vi "BLE_Module_EOL.vi"(8 "Error In":errorcluster, 9 "DUTBLEMACAddress":string="d8:3b:da:49:e3:cd", 10 "DUTBLEName":string="MyESP32", 11 "VISA resource name":refnum<visa-resource-name>) -> (0 "Error Out":errorcluster, 2 "FAIL":bool, 3 "PASS":bool, 5 "Read Status":string)   [LabVIEW 2025]
doc: "Simple string based state machine with internal error handling.\n\n--------------------\n<Author>\n<Company>"
uses:
  controls/TypeDefReadBuffer.ctl
  controls/BLE_States.ctl
  <vilib>/Utility/error.llb/Trim Whitespace One-Sided.vi
  <vilib>/Instr/_visa.llb/VISA Configure Serial Port (Instr).vi
panel:
  out "read_buffer":T1
  in  "Stop":bool
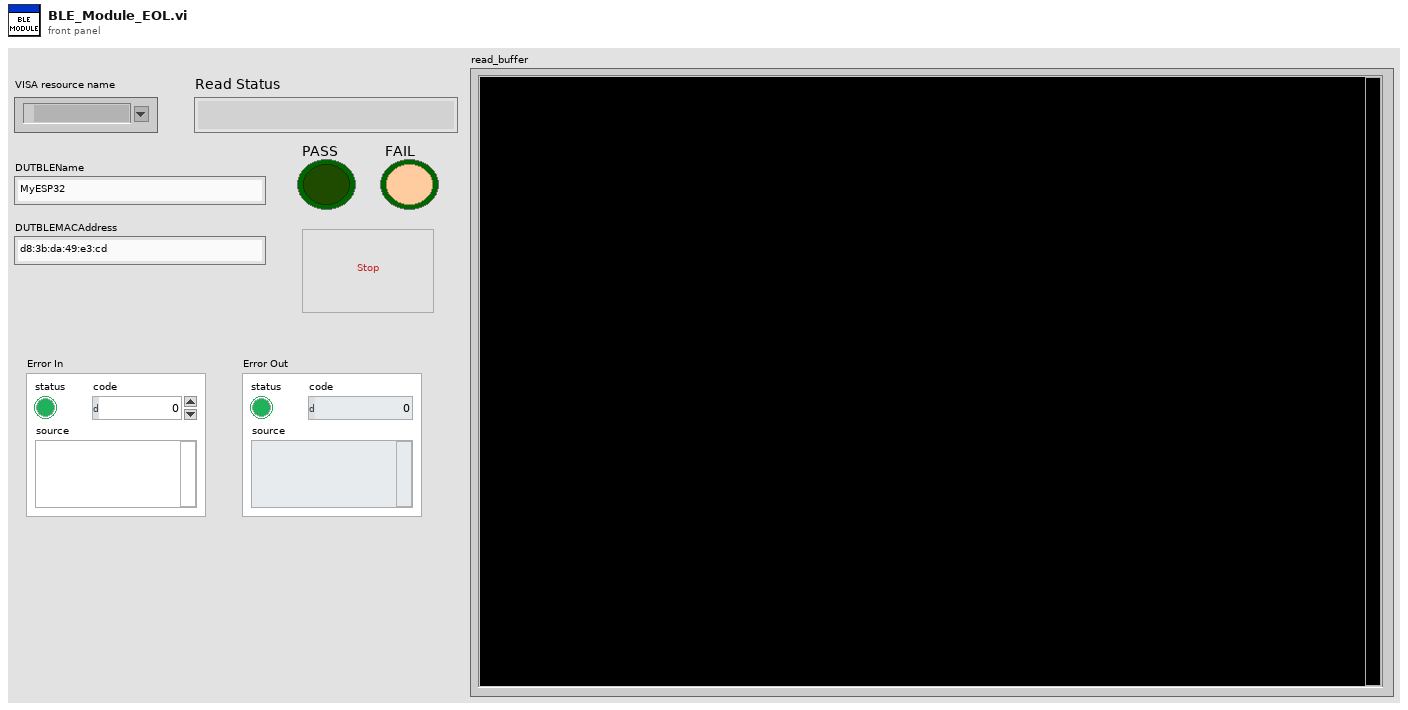
[diagram p1: front panel]
types:
  T1 = typedef "TypeDefReadBuffer.ctl" = string
  T2 = typedef "BLE_States.ctl" = enum16{"Init", "Init_BLE", "DUT_BLE_name", "DUT_BLE_macid", "scan", "ReadSerialContinously", "Disconnect_BLE", "Read_Disconnect_BLE", "Uninit_BLE", "Exit"}
  T3 = cluster{"Message":string, "VISA resource name":refnum<visa-resource-name>}
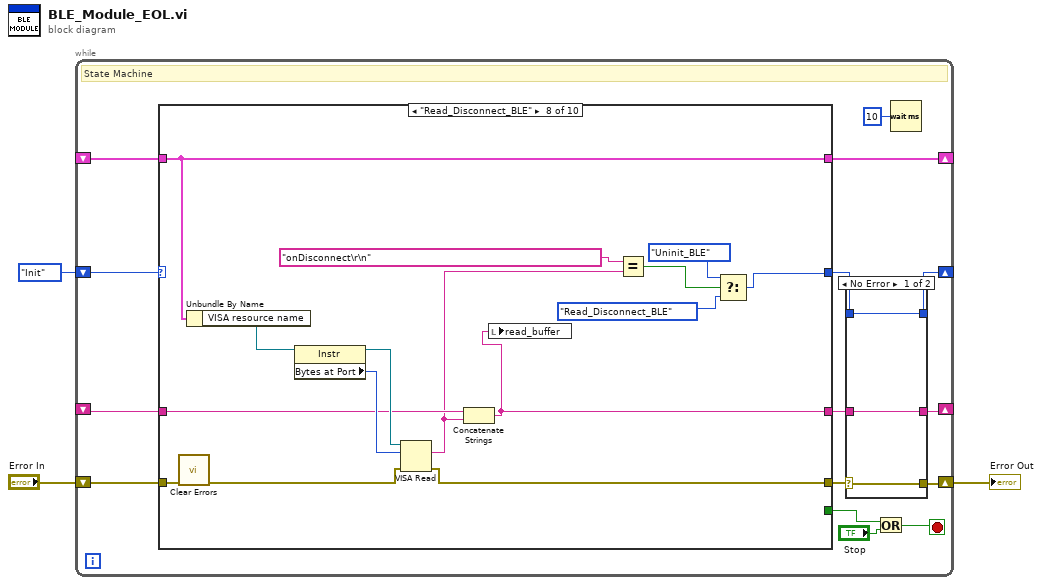
[diagram p0: block diagram]
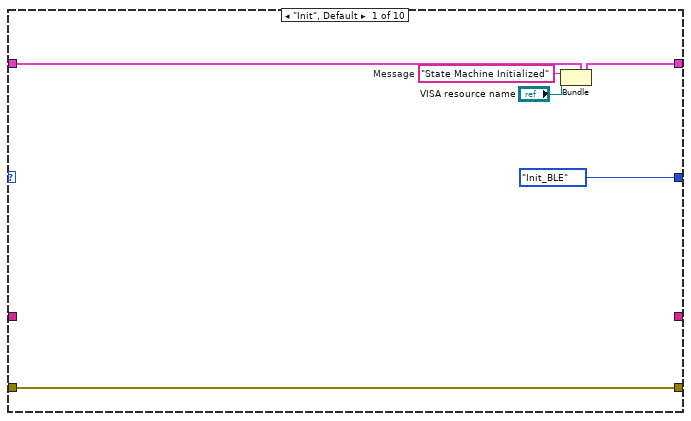
[diagram p2: hidden frame]
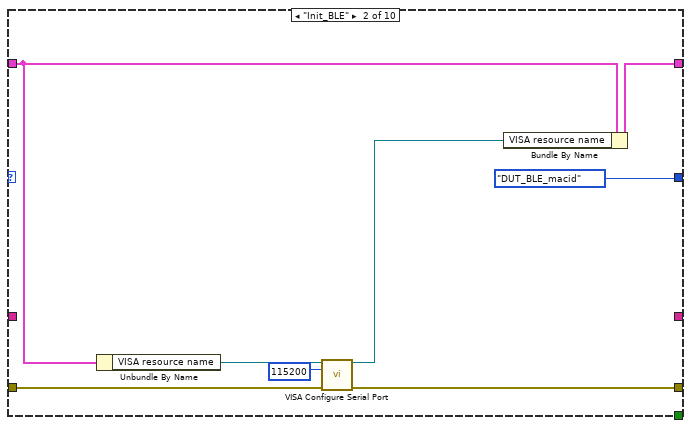
[diagram p3: hidden frame]
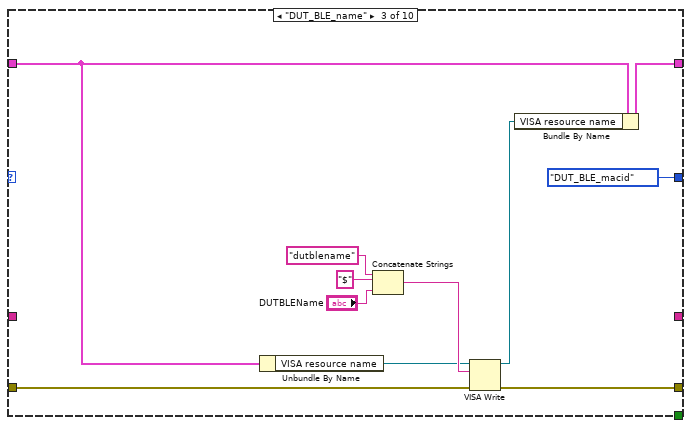
[diagram p4: hidden frame]
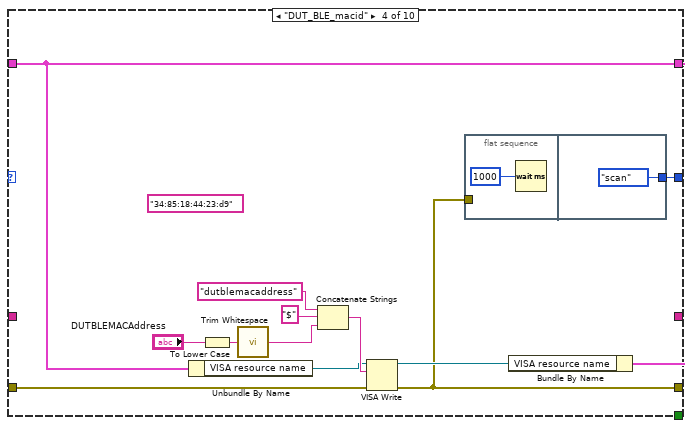
[diagram p5: hidden frame]
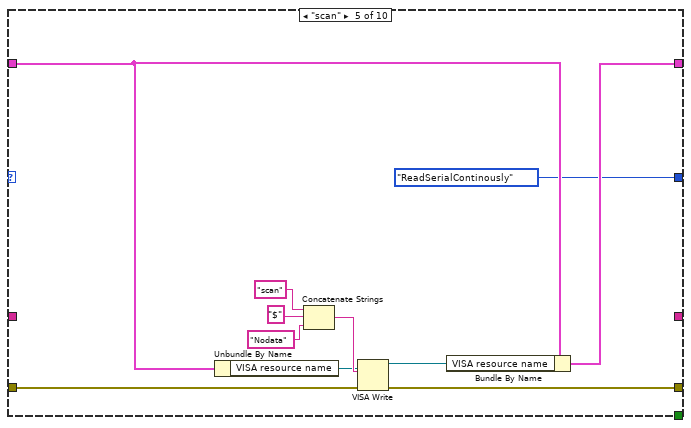
[diagram p6: hidden frame]
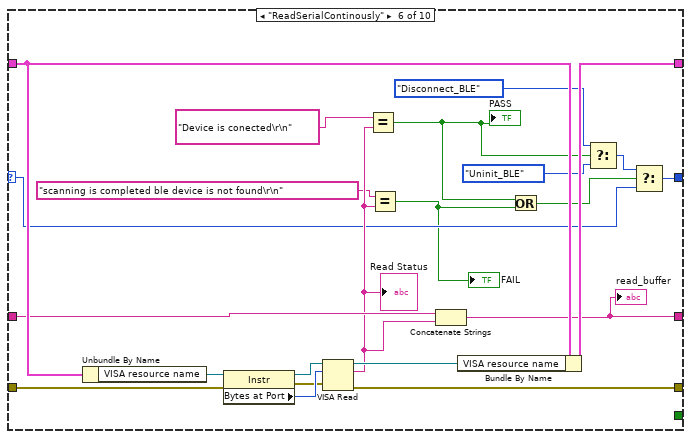
[diagram p7: hidden frame]
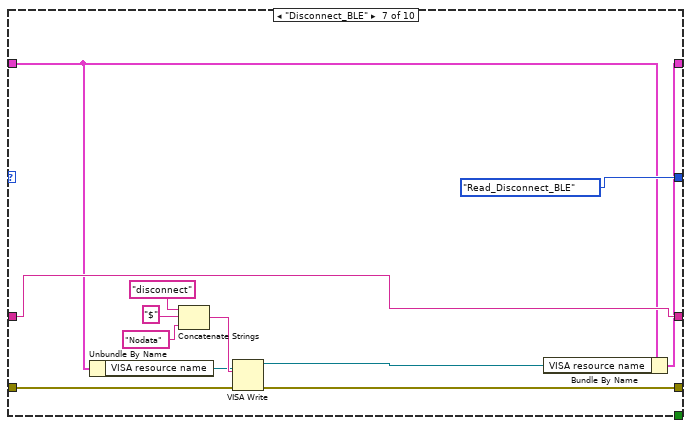
[diagram p8: hidden frame]
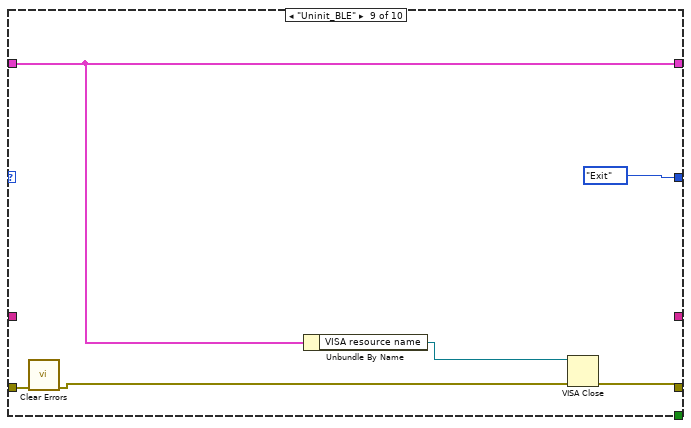
[diagram p9: hidden frame]
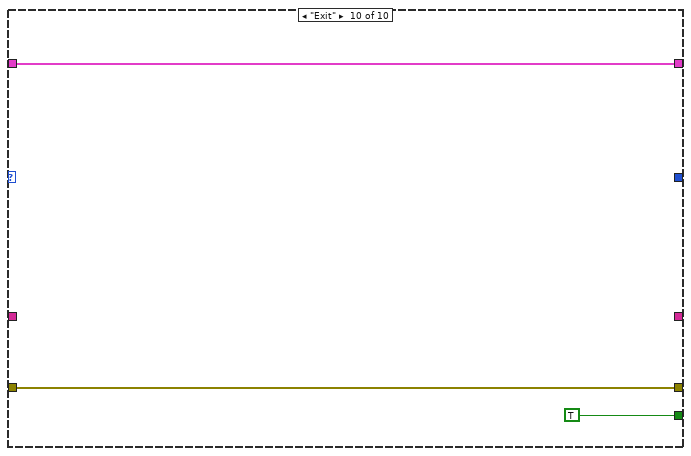
[diagram p10: hidden frame]
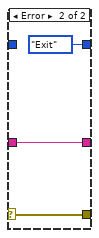
[diagram p11: hidden frame]
diagram:
  n1 = while {
    shift-right: [w11] -> _
    shift-left: BLE_States."Init" -> [w18]
    shift-right: [w16] -> _
    shift-left: _ -> [w17]
    shift-right: [w13] -> w3
    shift-left: "Error In" -> [w15]
    shift-right: [w5] -> _
    shift-left: _ -> [w6]
    stop <- w8 stop-if-true
    # "State Machine"
    n2 = case shown="\"Read_Disconnect_BLE\"" w18 {
      selector: w18 -> [_ _ _ _ _ w76 _ _ _ _]
      tunnel: w15 -> [w20 w31 w42 w54 w61 w87 w98 w117 w123 w125]
      tunnel: [w20 w30 w41 w47 w60 w91 w96 w110 w124 w125] -> w14
      tunnel: [_ _ _ _ _ _ _ _ _ TRUE] -> w9
      tunnel: [BLE_States."Init_BLE" BLE_States."DUT_BLE_macid" BLE_States."DUT_BLE_macid" w48 BLE_States."ReadSerialContinously" w81 BLE_States."Read_Disconnect_BLE" w107 BLE_States."Exit" _] -> w12
      tunnel: w17 -> [w21 w28 w36 w51 w63 w85 w94 w118 w120 w126]
      tunnel: [w23 w26 w34 w50 w62 w84 w92 w118 w120 w126] -> w16
      tunnel: w6 -> [_ _ _ _ _ w80 w95 w113 _ _]
      tunnel: [_ _ _ _ _ w79 w95 w112 _ _] -> w4
      frame "Init", Default {
        w24 = "State Machine Initialized"  # Message
        # "Initialize the state machine."
        n3 = Bundle(cluster=w21, "Message"=w24, "VISA resource name"="VISA resource name") -> (w23:T3)
      }
      frame "Init_BLE" {
        n4 = Unbundle By Name(w28) -> ("VISA resource name"=w29:refnum<visa-resource-name>)
        n5 = call-poly "VISA Configure Serial Port"("VISA resource name"=w29, "baud rate (9600)"=u32 115200, "error in (no error)"=w31) -> ("VISA resource name out"=w27:refnum<visa-resource-name>, "error out"=w30:errorcluster)  [unwired: 11 in]
        n6 = Bundle By Name(cluster=w28, "VISA resource name"=w27) -> (w26:T3)
      }
      frame "DUT_BLE_name" {
        n7 = Unbundle By Name(w36) -> ("VISA resource name"=w37:refnum<visa-resource-name>)
        n8 = Concatenate Strings("dutblename", "$" ("string"), "DUTBLEName") -> (w43:string)
        n9 = VISA Write(VISA resource name=w37, write buffer=w43, error in (no error)=w42) -> (VISA resource name out=w35:refnum<visa-resource-name>, error out=w41:errorcluster)  [unwired: 1 out]
        n10 = Bundle By Name(cluster=w36, "VISA resource name"=w35) -> (w34:T3)
      }
      frame "DUT_BLE_macid" {
        (unwired) "34:85:18:44:23:d9" ("DUTBLEMACAddress")
        n11 = Unbundle By Name(w51) -> ("VISA resource name"=w52:refnum<visa-resource-name>)
        n12 = To Lower Case(string="DUTBLEMACAddress") -> (all lower case string=w44:string)
        n13 = call <vilib>:"Trim Whitespace.vi"("string"=w44) -> ("trimmed string"=w45:string)  [unwired: 1 in]
        n14 = Concatenate Strings("dutblemacaddress", "$" ("string"), w45) -> (w53:string)
        n15 = VISA Write(VISA resource name=w52, write buffer=w53, error in (no error)=w54) -> (VISA resource name out=w49:refnum<visa-resource-name>, error out=w47:errorcluster)  [unwired: 1 out]
        n16 = flat-sequence {
          tunnel: w47 -> [_]
          tunnel: [BLE_States."scan"] -> w48
          frame #0 {
            n17 = Wait (ms)(milliseconds to wait=u32 1000) -> ()  [unwired: 1 out]
          }
          frame #1 {
          }
        }
        n18 = Bundle By Name(cluster=w51, "VISA resource name"=w49) -> (w50:T3)
      }
      frame "scan" {
        n19 = Unbundle By Name(w63) -> ("VISA resource name"=w65:refnum<visa-resource-name>)
        n20 = Concatenate Strings("scan", "$" ("string"), "Nodata" ("DUTBLEMACAddress 2")) -> (w66:string)
        n21 = VISA Write(VISA resource name=w65, write buffer=w66, error in (no error)=w61) -> (VISA resource name out=w64:refnum<visa-resource-name>, error out=w60:errorcluster)  [unwired: 1 out]
        n22 = Bundle By Name(cluster=w63, "VISA resource name"=w64) -> (w62:T3)
      }
      frame "ReadSerialContinously" {
        n23 = Unbundle By Name(w85) -> ("VISA resource name"=w90:refnum<visa-resource-name>)
        n24 = property class="Instr"(reference=w90, error in=w87) -> (reference out=w88:refnum<visa-resource-name>, error out=w86:errorcluster, "Bytes at Port"=w89:u32)
        n25 = VISA Read(VISA resource name=w88, byte count=w89, error in (no error)=w86) -> (VISA resource name out=w83:refnum<visa-resource-name>, read buffer=w78:string, error out=w91:errorcluster)  [unwired: 1 out]
        "Read Status" <- w78
        n26 = Equal?(x="Device is conected\r\n", y=w78) -> (x = y?=w71:bool)
        "PASS" <- w71
        n27 = Equal?(x="scanning is completed ble device is not found\r\n", y=w78) -> (x = y?=w70:bool)
        "FAIL" <- w70
        n28 = Concatenate Strings(w80, w78) -> (w79:string)
        "read_buffer" <- w79
        n29 = Bundle By Name(cluster=w85, "VISA resource name"=w83) -> (w84:T3)
        n30 = Or(x=w71, y=w70) -> (x .or. y?=w72:bool)
        n31 = Select(t=BLE_States."Disconnect_BLE", s=w71, f=BLE_States."Uninit_BLE" ("t")) -> (s? t:f=w73:T2)
        n32 = Select(t=w73, s=w72, f=w76) -> (s? t:f=w81:T2)
      }
      frame "Disconnect_BLE" {
        n33 = Unbundle By Name(w94) -> ("VISA resource name"=w99:refnum<visa-resource-name>)
        n34 = Concatenate Strings("disconnect", "$" ("string"), "Nodata" ("DUTBLEMACAddress 2")) -> (w100:string)
        n35 = VISA Write(VISA resource name=w99, write buffer=w100, error in (no error)=w98) -> (VISA resource name out=w93:refnum<visa-resource-name>, error out=w96:errorcluster)  [unwired: 1 out]
        n36 = Bundle By Name(cluster=w94, "VISA resource name"=w93) -> (w92:T3)
      }
      frame "Read_Disconnect_BLE" {
        # "Exit the State Machine"
        n37 = call <vilib>:"Clear Errors.vi"("error in (no error)"=w117) -> ("error out"=w111:errorcluster)  [unwired: 5 in, 1 out]
        n38 = Unbundle By Name(w118) -> ("VISA resource name"=w116:refnum<visa-resource-name>)
        n39 = property class="Instr"(reference=w116) -> (reference out=w115:refnum<visa-resource-name>, "Bytes at Port"=w114:u32)  [unwired: 1 in, 1 out]
        n40 = VISA Read(VISA resource name=w115, byte count=w114, error in (no error)=w111) -> (read buffer=w108:string, error out=w110:errorcluster)  [unwired: 2 out]
        n41 = Concatenate Strings(w113, w108) -> (w112:string)
        n42 = local write "read_buffer"(w112) -> ()
        n43 = Equal?(x="onDisconnect\r\n", y=w108) -> (x = y?=w106:bool)
        n44 = Select(t=BLE_States."Uninit_BLE", s=w106, f=BLE_States."Read_Disconnect_BLE") -> (s? t:f=w107:T2)
      }
      frame "Uninit_BLE" {
        # "Exit the State Machine"
        n45 = call <vilib>:"Clear Errors.vi"("error in (no error)"=w123) -> ("error out"=w122:errorcluster)  [unwired: 5 in, 1 out]
        n46 = Unbundle By Name(w120) -> ("VISA resource name"=w119:refnum<visa-resource-name>)
        n47 = VISA Close(VISA resource name=w119, error in (no error)=w122) -> (error out=w124:errorcluster)
      }
      frame "Exit" {
        # "Exit the State Machine"
      }
    }
    n48 = case shown="No Error" w14 {
      selector: w14 -> [w130 w133]
      tunnel: [w130 w133] -> w13
      tunnel: w12 -> [w129 _]
      tunnel: [w129 BLE_States."Exit"] -> w11
      tunnel: [w128 w131] -> w5
      tunnel: w4 -> [w128 w131]
      frame No Error {
      }
      frame Error {
      }
    }
    n49 = Or(x=w9, y="Stop") -> (x .or. y?=w8:bool)
    n50 = Wait (ms)(milliseconds to wait=u32 10) -> ()  [unwired: 1 out]
  }
  "Error Out" <- w3
